vi "Write FIFO.vi"(8 "error in (no error)":errorcluster, 10 "FIFO":bool, 11 "NI_AWS_SQS in":refnum<class "Queue.lvclass">) -> (0 "error out":errorcluster, 3 "NI_AWS_SQS out":refnum<class "Queue.lvclass">)   [LabVIEW 2015, in "NI_AWS_SQS.lvlib" / "Queue.lvclass"]
uses:
  Queue.lvclass
  Queue.lvclass/Queue.ctl
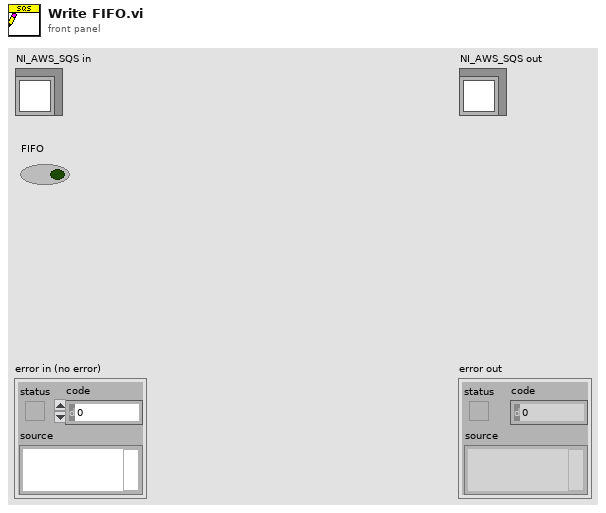
[diagram p1: front panel]
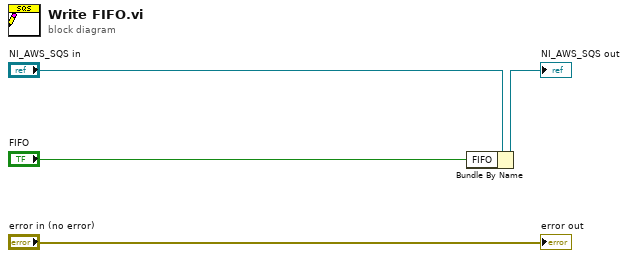
[diagram p0: block diagram]
diagram:
  n1 = Bundle By Name(cluster="NI_AWS_SQS in", "FIFO"="FIFO") -> (→"NI_AWS_SQS out":refnum<class "Queue.lvclass">)
  "error out" <- "error in (no error)"
